vi "Convert Channel Values to Quadrature Encoder Measure Digital Settings.vi"(9 "Length":i32, 10 "Index":i32, 11 "Channel Values in":dbl[](array[numeric])) -> (2 "Quadrature Encoder Measure Digital Settings":T1, 3 "Channel Values out":dbl[](array[numeric]))   [LabVIEW 2018, in "FPGA Addon Engine.lvlib"]
uses:
  FPGA Addon Engine.lvlib
  Submodules/Source/Types/QuadratureEncoder.Measure.Digital.Settings.ctl
  Submodules/Source/Speciality FPGA IO.lvlib
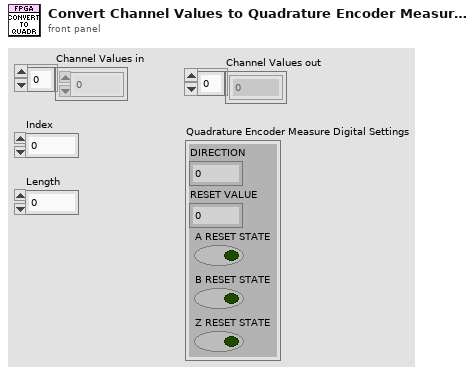
[diagram p1: front panel]
types:
  T1 = typedef "Speciality FPGA IO.lvlib/QuadratureEncoder.Measure.Digital.Settings.ctl" = cluster{"DIRECTION":u8, "RESET VALUE":i32, "A RESET STATE":bool, "B RESET STATE":bool, "Z RESET STATE":bool}
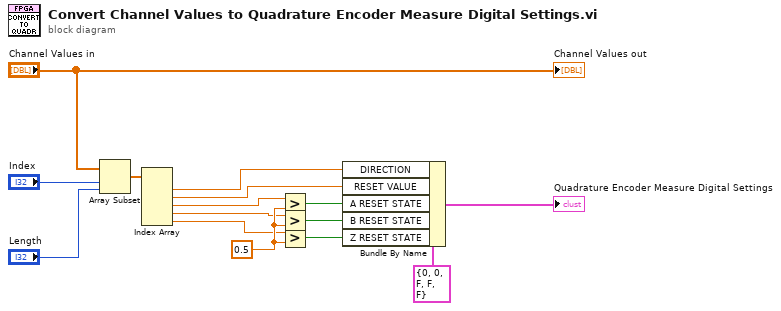
[diagram p0: block diagram]
diagram:
  w7 = 0.5 ("y")
  n1 = Array Subset(array="Channel Values in", index="Index", length="Length") -> (w1:dbl[])
  n2 = Index Array(array=w1) -> (element #1=w10:dbl, element #2=w9:dbl, element #3=w6:dbl, element #4=w5:dbl, element #5=w4:dbl)  [unwired: 5 in]
  n3 = Greater?(x=w6, y=w7) -> (0:w8:bool)
  n4 = Greater?(x=w5, y=w7) -> (0:w3:bool)
  n5 = Greater?(x=w4, y=w7) -> (0:w2:bool)
  n6 = Bundle By Name(cluster=T1 {"DIRECTION"=0, "RESET VALUE"=0, "A RESET STATE"=FALSE, "B RESET STATE"=FALSE, "Z RESET STATE"=FALSE} ("Settings"), "DIRECTION"=w10, "RESET VALUE"=w9, "A RESET STATE"=w8, "B RESET STATE"=w3, "Z RESET STATE"=w2) -> (→"Quadrature Encoder Measure Digital Settings":T1)
  "Channel Values out" <- "Channel Values in"
